vi "Write ITX (XY).vi"(4 "Commands":string, 6 "Notes":string, 8 "error in":errorcluster, 9 "wavenames":string[](array[string]), 10 "XY Array":cluster{"X  array":dbl[], "Y  Array":dbl[]}[](array[cluster]), 11 "filename":path) -> (0 "error out":errorcluster, 3 "file":path)   [LabVIEW 2019, in "LV-Data.ITX.lvclass"]
uses:
  LV-Data.ITX.lvclass
panel:
  out "String":string
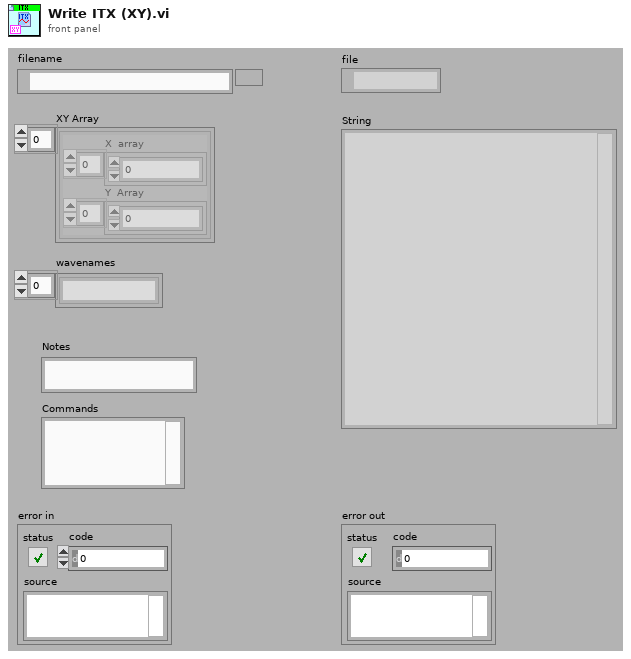
[diagram p1: front panel]
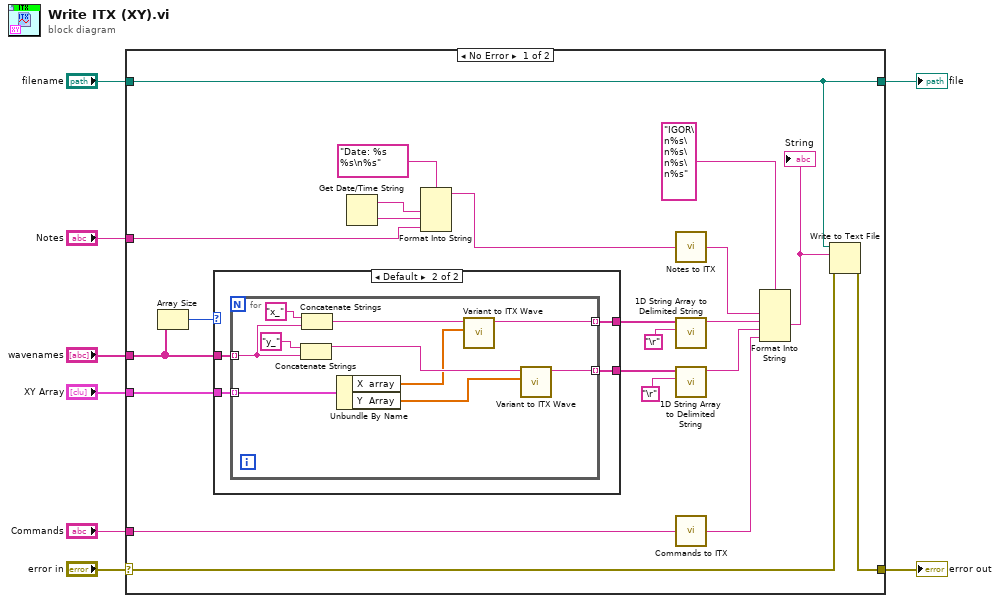
[diagram p0: block diagram]
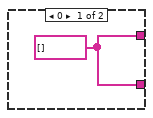
[diagram p2: hidden frame]
diagram:
  n1 = case shown="No Error" "error in" {
    selector: "error in" -> [w25 w47]
    tunnel: "filename" -> [w26 w46]
    tunnel: "wavenames" -> [w30 _]
    tunnel: "Notes" -> [w9 _]
    tunnel: "XY Array" -> [w28 _]
    tunnel: [w27 w47] -> w4
    tunnel: [w26 w46] -> w2
    tunnel: "Commands" -> [w24 _]
    frame No Error {
      n2 = Array Size(array=w30) -> (size(s)=w29:i32)
      n3 = case shown="Default" w29 {
        tunnel: w30 -> [_ w35]
        tunnel: w28 -> [_ w34]
        tunnel: [w31 w33] -> w17
        tunnel: [w31 w32] -> w16
        frame 0 {
          w31 = string[] []
        }
        frame Default {
          n4 = for {
            tunnel: [w36] -> w33 mode=indexing
            tunnel: w35 -> [w42] mode=indexing
            tunnel: w34 -> [w43] mode=indexing
            tunnel: [w37] -> w32 mode=indexing
            n5 = Concatenate Strings("y_" ("string"), w42) -> (w40:string)
            n6 = Concatenate Strings("x_" ("string"), w42) -> (w41:string)
            n7 = Unbundle By Name(w43) -> ("X  array"=w39:dbl[], "Y  Array"=w38:dbl[])
            n8 = call "Variant to ITX Wave.vi"("2D Array"=w39, "Wavename"=w41) -> ("ITX Wave"=w36:string)  [unwired: 8 in, 1 out]
            n9 = call "Variant to ITX Wave.vi"("2D Array"=w38, "Wavename"=w40) -> ("ITX Wave"=w37:string)  [unwired: 8 in, 1 out]
          }
        }
      }
      n10 = Get Date/Time String() -> (date string=w22:string, time string=w23:string)  [unwired: 3 out]
      n11 = Format Into String(format string="Date: %s %s\n%s", w22, w23, w9) -> (resulting string=w18:string)  [unwired: 2 in, 1 out]
      n12 = call "Notes to ITX.vi"("Notes"=w18) -> ("ITX Notes"=w11:string)
      n13 = call <vilib>:"1D String Array to Delimited String.vi"("delimiter"="\r", "string array"=w17) -> ("delimited string"=w13:string)  [unwired: 9 in]
      n14 = call <vilib>:"1D String Array to Delimited String.vi"("delimiter"="\r", "string array"=w16) -> ("delimited string"=w12:string)  [unwired: 9 in]
      n15 = call "Commands to ITX.vi"("Commands"=w24) -> ("ITX Commands"=w10:string)
      n16 = Format Into String(format string="IGOR\n%s\n%s\n%s\n%s", w11, w13, w12, w10) -> (resulting string=w19:string)  [unwired: 2 in, 1 out]
      "String" <- w19
      n17 = Write to Text File(file (use dialog)=w26, text=w19, error in=w25) -> (error out=w27:errorcluster)  [unwired: 3 out]
    }
    frame Error {
    }
  }
  "file" <- w2
  "error out" <- w4
